vi "Write Static On.vi"(8 "error in (no error)":errorcluster, 10 "Static On":bool, 11 "Meerstetter output in":refnum<class "Meerstetter output.lvclass">) -> (0 "error out":errorcluster, 3 "Meerstetter output out":refnum<class "Meerstetter output.lvclass">)   [LabVIEW 2014, in "Meerstetter Lib.lvlib" / "Meerstetter output.lvclass"]
uses:
  Meerstetter output.lvclass
  Meerstetter output.lvclass/Meerstetter output.ctl
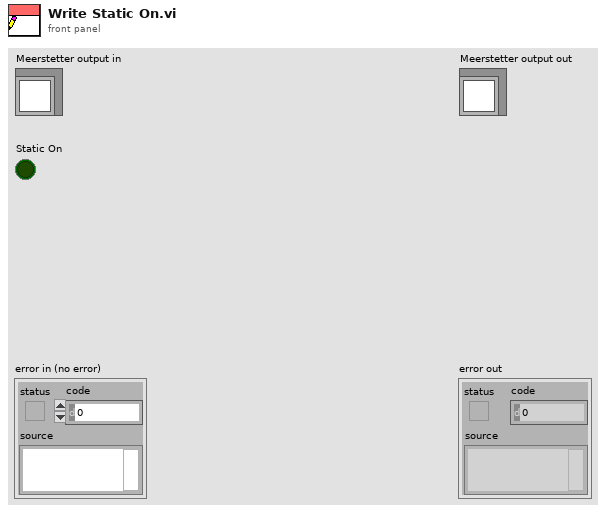
[diagram p1: front panel]
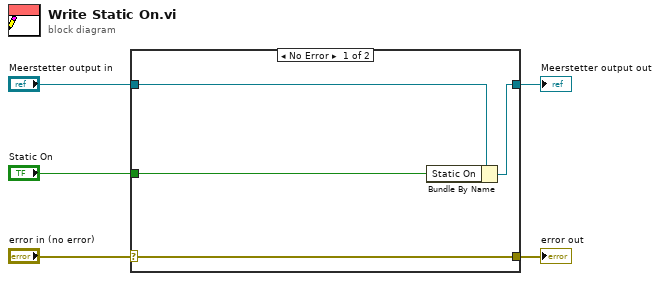
[diagram p0: block diagram]
diagram:
  n1 = case shown="No Error" "error in (no error)" {
    selector: "error in (no error)" -> [w9 w10]
    tunnel: [w9 w10] -> w4
    tunnel: [w7 w11] -> w2
    tunnel: "Meerstetter output in" -> [w8 w11]
    tunnel: "Static On" -> [w6 _]
    frame No Error {
      n2 = Bundle By Name(cluster=w8, "Static On"=w6) -> (w7:refnum<class "Meerstetter output.lvclass">)
    }
    frame Error {
    }
  }
  "error out" <- w4
  "Meerstetter output out" <- w2
